vi "test_abs_activity_vapor.vi"() -> ()   [LabVIEW 2017]
doc: "Minimal example that demonstrates functions implemented in the SorpPropLib for absorption working pairs based on the activity approach and using the vapor pressure as additional property."
panel:
  in  "Molar volume of second component in m3/mol (Input)":dbl=-1.0
  in  "Molar volume of first component in m3/mol (Input)":dbl=-1.0
  out "Pressure":cluster{dbl[], dbl[]}[](graph)=[{[500000.0, 500001.0, 500002.0, 500003.0, 500004.0, 500005.0, 500006.0, 500007.0, 500008.0, 500009.0, 500010.0, 500011.0, 500012.0, 500013.0, 500014.0, 500015.0, 500016.0, 500017.0, 500018.0, 500019.0, 500020.0, 500021.0, 500022.0, 500023.0, 500024.0], [500000.0, 500001.00000000006, 500002.00000000006, 500003.0000000001, 500004.00000000006, 500005.0, 500006.0000000001, 500007.0, 500008.0, 500008.9999999998, 500010.0000000002, 500011.0, 500012.0, 500012.9999999999, 500013.9999999999, 500015.0000000001, 500015.99999999994, 500017.0000000001, 500018.0000000001, 500018.9999999998, 500019.9999999999, 500021.0000000001, 500022.0, 500023.0, 500024.0]}]
  out "Mole fraction in liquid phase":cluster{dbl[], dbl[]}[](graph)=[{[500000.0, 500001.0, 500002.0, 500003.0, 500004.0, 500005.0, 500006.0, 500007.0, 500008.0, 500009.0, 500010.0, 500011.0, 500012.0, 500013.0, 500014.0, 500015.0, 500016.0, 500017.0, 500018.0, 500019.0, 500020.0, 500021.0, 500022.0, 500023.0, 500024.0], [0.2190016642998693, 0.219002568669402, 0.21900347304349513, 0.2190043774221486, 0.21900528180536258, 0.21900618619313716, 0.21900709058547257, 0.21900799498236828, 0.21900889938382498, 0.21900980378984214, 0.2190107082004204, 0.21901161261555932, 0.2190125170352591, 0.21901342145951969, 0.21901432588834138, 0.21901523032172426, 0.2190161347596678, 0.21901703920217264, 0.21901794364923868, 0.21901884810086555, 0.21901975255705397, 0.21902065701780365, 0.21902156148311439, 0.21902246595298647, 0.21902337042742026]}]
  in  "WorkingPair (Input)":T1={"no_iso"=1, "no_p_sat"=1, "path_db"="D:\\Driesel\\SorpLibLocal\\labview_wrapper\\data\\json\\sorpproplib.json", "wp_as"="lubricant", "wp_st"="POE", "wp_iso"="WilsonFixedDl", "wp_rf"="R-134a", "rf_rhol"="SaturatedLiquidDensity_EoS1", "no_rhol"=1, "rf_psat"="VaporPressure_EoS1"}
  in  "Temperature in K (Input)":dbl=300.0
  in  "Pressure in Pa (Input)":dbl=500000.0
  # "Increase pressure by 25 Pa in steps of 1 Pa."
  # "Selecting -1: Constant molar volumes stored in data base are used for calculations!"
  # "Path to database"
  # "Name of sorbent"
  # "Name of sub-type of sorbent"
  # "Name of refrigerant"
  # "Name of isotherm"
  # "ID of isotherm"
  # "Name of calculation approach for vapor pressure"
  # "ID of vapor pressure equation"
  # "Name of calculation approach for liquid density"
  # "ID of liquid density equation"
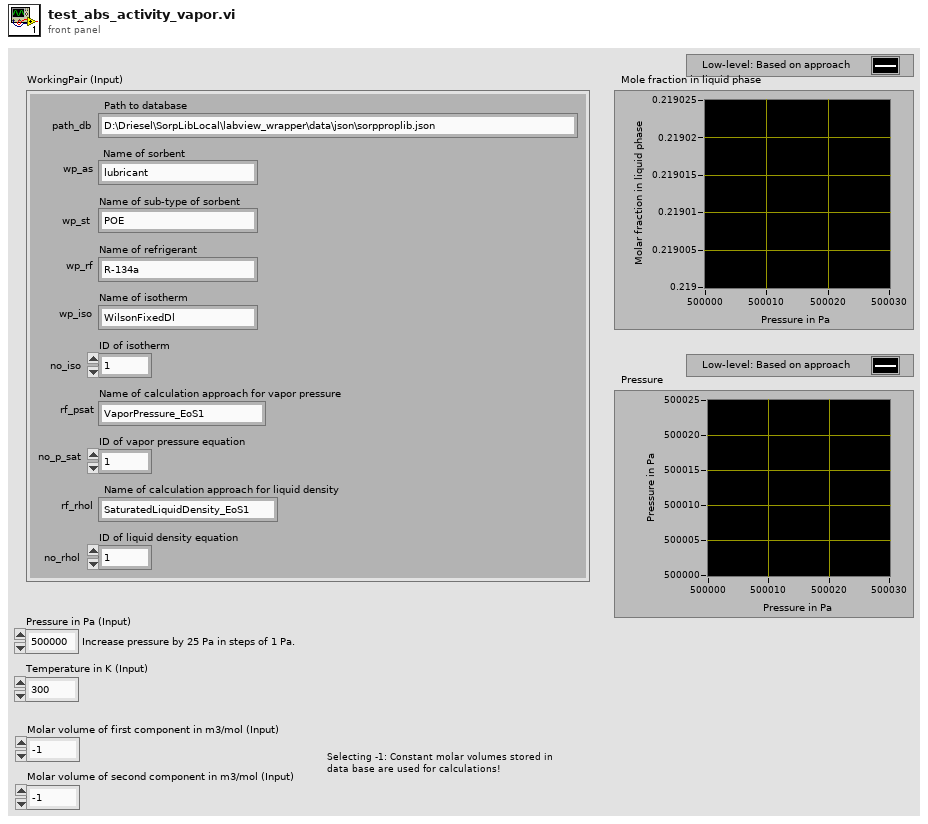
[diagram p1: front panel]
types:
  T1 = cluster{"no_iso":i32, "no_p_sat":i32, "path_db":string, "wp_as":string, "wp_st":string, "wp_iso":string, "wp_rf":string, "rf_rhol":string, "no_rhol":i32, "rf_psat":string}
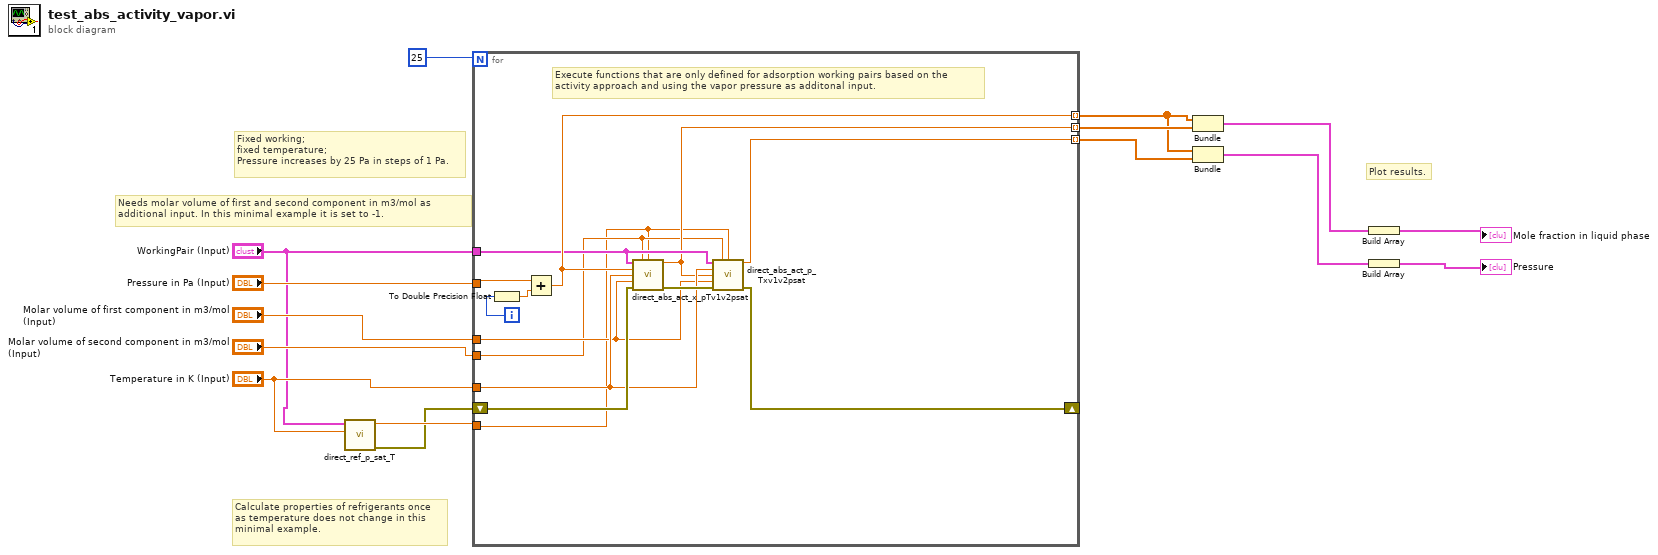
[diagram p0: block diagram]
diagram:
  # "Needs molar volume of first and second component in m3/mol as \nadditional input. In this minimal example it is set to -1."
  # "Calculate properties of refrigerants once\nas temperature does not change in this\nminimal example."
  # "Plot results."
  # "Fixed working;\nfixed temperature;\nPressure increases by 25 Pa in steps of 1 Pa."
  n1 = call "direct_ref_p_sat_T.vi"("Temperature in K (Input)"="Temperature in K (Input)", "WorkingPair (Input)"="WorkingPair (Input)") -> ("Error (Output)"=w2:errorcluster, "Saturation pressure in Pa (Output)"=w4:dbl)  [unwired: 8 in]
  n2 = for {
    N: 25 -> [_]
    tunnel: "Pressure in Pa (Input)" -> [w29]
    tunnel: "Temperature in K (Input)" -> [w20]
    tunnel: "WorkingPair (Input)" -> [w21]
    shift-right: [w23] -> _
    shift-left: w2 -> [w25]
    tunnel: [w26] -> w12 mode=indexing
    tunnel: [w19] -> w13 mode=indexing
    tunnel: [w22] -> w11 mode=indexing
    tunnel: "Molar volume of first component in m3/mol (Input)" -> [w18]
    tunnel: w4 -> [w16]
    tunnel: "Molar volume of second component in m3/mol (Input)" -> [w17]
    i -> [w28]
    # "Execute functions that are only defined for adsorption working pairs based on the\nactivity approach and using the vapor pressure as additonal input."
    n3 = To Double Precision Float(number=w28) -> (double precision float=w27:dbl)
    n4 = Add(x=w29, y=w27) -> (x+y=w26:dbl)
    n5 = call "direct_abs_act_x_pTv1v2psat.vi"("WorkingPair (Input)"=w21, "Molar volume of second component in m3/mol (Input)"=w17, "Saturation pressure of first component in Pa (Input)"=w16, "Pressure in Pa (Input)"=w26, "Temperature in K (Input)"=w20, "Molar volume of first component in m3/mol (Input)"=w18, "Error (Input)"=w25) -> ("Mole fraction in liquid phase in mol/mol(Output)"=w19:dbl, "Error (Output)"=w24:errorcluster)  [unwired: 7 in]
    n6 = call "direct_abs_act_p_Txv1v2psat.vi"("WorkingPair (Input)"=w21, "Molar volume of second component in m3/mol (Input)"=w17, "Saturation pressure of first component in Pa (Input)"=w16, "Temperature in K (Input)"=w20, "Mole fraction in liquid phase in mol/mol (Input)"=w19, "Molar volume of first component in m3/mol (Input)"=w18, "Error (Input)"=w24) -> ("Pressure in Pa (Output)"=w22:dbl, "Error (Output)"=w23:errorcluster)  [unwired: 7 in]
  }
  n7 = Bundle(w12, w13) -> (w10:cluster{dbl[], dbl[]})  [unwired: 1 in]
  n8 = Bundle(w12, w11) -> (w9:cluster{dbl[], dbl[]})  [unwired: 1 in]
  n9 = Build Array(w10) -> (→"Mole fraction in liquid phase":cluster{dbl[], dbl[]}[])
  n10 = Build Array(w9) -> (→"Pressure":cluster{dbl[], dbl[]}[])
